vi "Write Status_timeout.vi"(8 "error in (no error)":errorcluster, 9 "TCS_timeout":bool, 10 "Status_timeout":bool, 11 "S4ACS_GUI in":refnum<class "S4ACS_GUI.lvclass">) -> (0 "error out":errorcluster, 3 "S4ACS_GUI out":refnum<class "S4ACS_GUI.lvclass">)   [LabVIEW 2018, in "S4ACS_GUI.lvclass"]
uses:
  S4ACS_GUI.lvclass
  S4ACS_GUI.lvclass/S4ACS_GUI.ctl
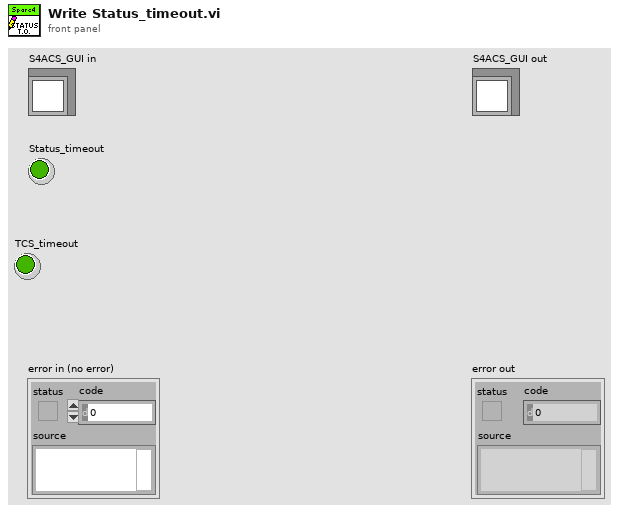
[diagram p1: front panel]
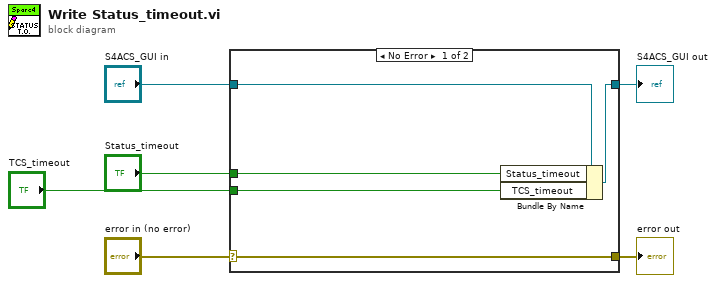
[diagram p0: block diagram]
diagram:
  n1 = case shown="No Error" "error in (no error)" {
    selector: "error in (no error)" -> [w11 w12]
    tunnel: [w11 w12] -> w5
    tunnel: [w9 w13] -> w3
    tunnel: "S4ACS_GUI in" -> [w10 w13]
    tunnel: "Status_timeout" -> [w8 _]
    tunnel: "TCS_timeout" -> [w7 _]
    frame No Error {
      n2 = Bundle By Name(cluster=w10, "Status_timeout"=w8, "TCS_timeout"=w7) -> (w9:refnum<class "S4ACS_GUI.lvclass">)
    }
    frame Error {
    }
  }
  "error out" <- w5
  "S4ACS_GUI out" <- w3
